vi "GetFontsWindows__FD__LCR.vi"(8 "error in (no error)":errorcluster) -> (0 "error out":errorcluster, 3 "Fonts":string[](array[string]))   [LabVIEW 2011]
doc: "SystemFonts.vi\n\nThis VI reads the windows registry to determine the installed system fonts. Having read the system fonts, the VI filters the font names and assign one to an indicator through a property node."
uses:
  <vilib>/registry/registry.llb/Registry RtKey.ctl
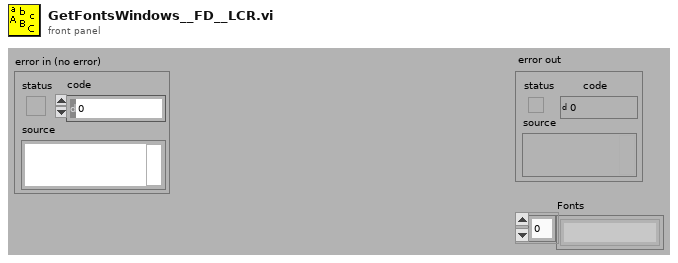
[diagram p1: front panel]
types:
  T1 = typedef "Registry RtKey.ctl" = enum32{"HKEY_CLASSES_ROOT", "HKEY_CURRENT_USER", "HKEY_LOCAL_MACHINE", "HKEY_USERS", "HKEY_PERFORMANCE_DATA", "HKEY_CURRENT_CONFIG", "HKEY_DYN_DATA"}
  T2 = typedef "Registry refnum.ctl" = refnum<k1>
  T3 = cluster{"numValues":i32, "maxValueNameLen":i32, "maxValueDataLen":i32}
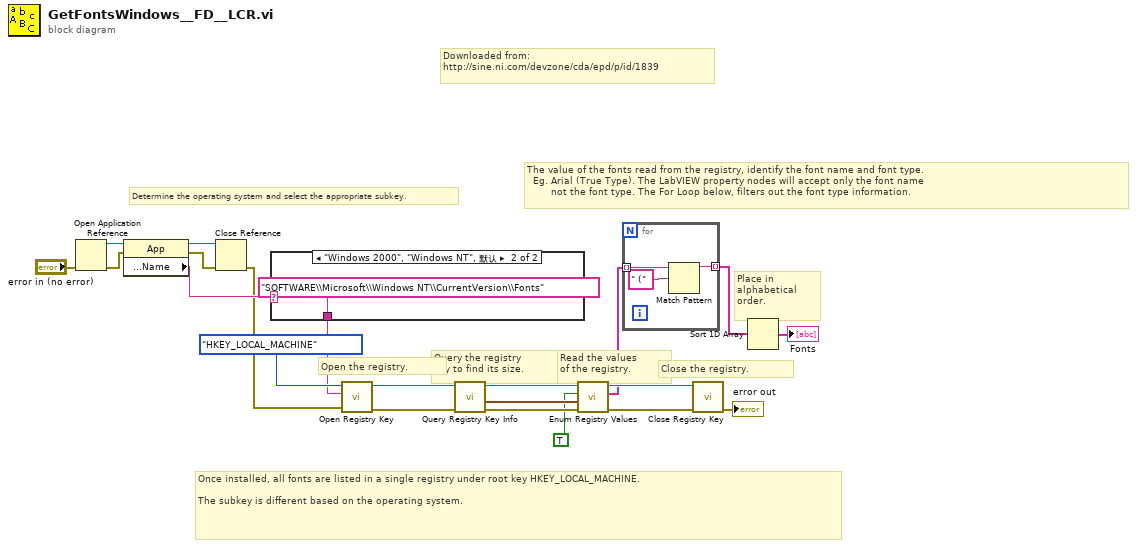
[diagram p0: block diagram]
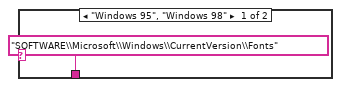
[diagram p2: hidden frame]
diagram:
  # "Downloaded from:\nhttp://sine.ni.com/devzone/cda/epd/p/id/1839"
  # "Determine the operating system and select the appropriate subkey."
  # "Place in \nalphabetical\norder."
  # "The value of the fonts read from the registry, identify the font name and font type. \n  Eg. Arial (True Type). The LabVIEW property nodes will accept only the font name\n        not the font type. The For Loop below, filters out the font type information."
  # "Close the registry."
  # "Query the registry \nkey to find its size."
  # "Open the registry."
  # "Read the values \nof the registry."
  # "Once installed, all fonts are listed in a single registry under root key HKEY_LOCAL_MACHINE.\n\nThe subkey is different based on the operating system."
  n1 = Open Application Reference(8:"error in (no error)") -> (0:w9:errorcluster, 3:w10:refnum<vi>)  [unwired: 3 in]
  n2 = property class="App"(reference=w10, error in=w9) -> (reference out=w5:refnum<vi>, error out=w6:errorcluster, "Operating System:Name"=w8:string)
  n3 = Close Reference(reference=w5, error in (no error)=w6) -> (error out=w4:errorcluster)
  n4 = case shown="\"Windows 2000\", \"Windows NT\", 默认" w8 {
    tunnel: ["SOFTWARE\\Microsoft\\Windows\\CurrentVersion\\Fonts" ("subkey") "SOFTWARE\\Microsoft\\Windows NT\\CurrentVersion\\Fonts" ("subkey")] -> w7
    frame "Windows 95", "Windows 98" {
    }
    frame "Windows 2000", "Windows NT", Default {
    }
  }
  n5 = call <vilib>:"Open Registry Key.vi"("error in (no error)"=w4, "subkey"=w7, "root key (HKEY_LOCAL_MACHINE)"=Registry_RtKey."HKEY_LOCAL_MACHINE") -> ("error out"=w20:errorcluster, "refnum out"=w19:T2)  [unwired: 7 in]
  n6 = call <vilib>:"Query Registry Key Info.vi"("error in (no error)"=w20, "refnum"=w19) -> ("error out"=w16:errorcluster, "value info"=w17:T3, "refnum out"=w18:T2)  [unwired: 5 in, 2 out]
  n7 = call <vilib>:"Enum Registry Values.vi"("error in (no error)"=w16, "value info"=w17, "retrieve data? (F)"=TRUE, "refnum"=w18) -> ("error out"=w14:errorcluster, "values"=w13:string[], "refnum out"=w15:T2)  [unwired: 2 in, 3 out]
  n8 = for {
    tunnel: w13 -> [w26] mode=indexing
    tunnel: [w25] -> w12 mode=indexing
    n9 = Match Pattern(string=w26, regular expression=" (") -> (before substring=w25:string)  [unwired: 1 in, 3 out]
  }
  n10 = call <vilib>:"Close Registry Key.vi"("error in (no error)"=w14, "refnum"=w15) -> ("error out"=→"error out":errorcluster)  [unwired: 5 in]
  n11 = Sort 1D Array(array=w12) -> (sorted array=→"Fonts":string[])
